vi "Util_DispWaypoint_Eng_To_SI.vi"(11 "WayPoints":T1[](array[typedef]) {"ANGLE" format="%13.3f"; "Y" format="%13.3f"; "X" format="%13.3f"}) -> (3 "WayPoints":T1[](array[typedef]) {"ANGLE" format="%13.3f"; "Y" format="%13.3f"; "X" format="%13.3f"})   [LabVIEW 2019, in "Trajectory_Library.lvlib"]
doc: "Utility function to convert utility waypoints from Inches, degrees to meters, radians. All the normal trajectory functions expect the units to be in meters, radians (unless otherwise specified)."
uses:
  Trajectory_Library.lvlib
  TypeDef/DISPLAY_WAYPOINT.ctl
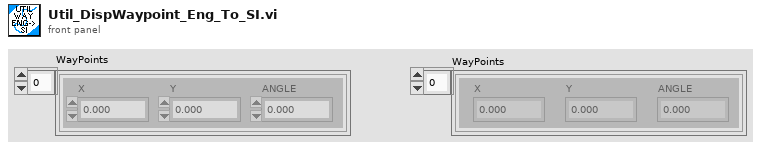
[diagram p1: front panel]
types:
  T1 = typedef "Trajectory_Library.lvlib/DISPLAY_WAYPOINT.ctl" = cluster{"X":dbl, "Y":dbl, "ANGLE":dbl}
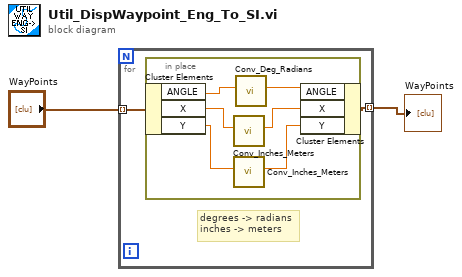
[diagram p0: block diagram]
diagram:
  n1 = for {
    tunnel: "WayPoints" -> [w4] mode=indexing
    tunnel: [w3] -> w1 mode=indexing
    # "degrees -> radians\ninches -> meters"
    n2 = in-place {
      n3 = in-place-cluster #1(w4) -> ("ANGLE"=w5:dbl, "X"=w10:dbl, "Y"=w8:dbl)
      n4 = call "Conv_Inches_Meters.vi"("INCH"=w10) -> ("Meters"=w9:dbl)  [unwired: 10 in]
      n5 = call "Conv_Inches_Meters.vi"("INCH"=w8) -> ("Meters"=w7:dbl)  [unwired: 10 in]
      n6 = call "Conv_Deg_Radians.vi"("Degress"=w5) -> ("Radians"=w6:dbl)  [unwired: 10 in]
      n7 = in-place-cluster #1("ANGLE"=w6, "X"=w9, "Y"=w7) -> (w3:T1)
    }
  }
  "WayPoints" <- w1
